vi "FSM Localization.vi"(0 "Signals":T2, 2 "Pressure Controls":T5, 4 "Dialog Indicator":refnum<vi>, 5 "error in (no error)":errorcluster, 6 "Manipulator Dynamics":refnum<vi>, 7 "Unblockage Parameters":T1, 8 "Pressure Levels [KPa]":refnum<vi>, 9 "Test and Offset Controls":T4, 10 "Test Signal Levels":refnum<vi>, 11 "Manipulator Controllers":T3, 13 "Abort":refnum<vi>) -> (15 "Aborted":bool, 16 "Blocked":bool, 19 "error out":errorcluster)   [LabVIEW 2012, in "Autopatcher Daemon.lvlib"]
uses:
  Autopatcher Daemon.lvlib
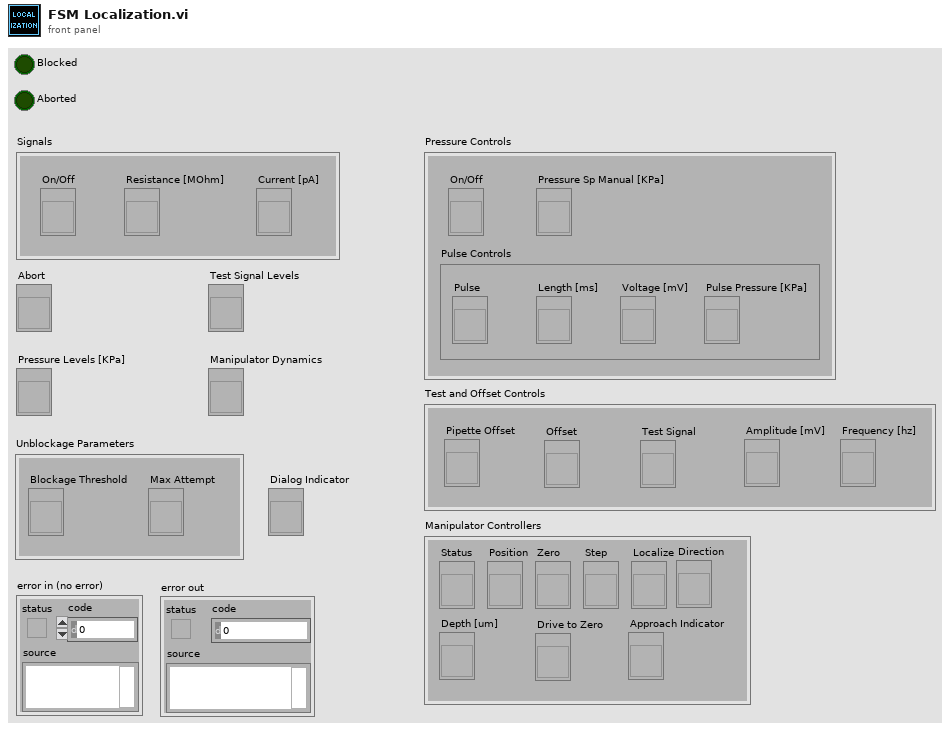
[diagram p1: front panel]
types:
  T1 = cluster{"Blockage Threshold":refnum<vi>, "Max Attempt":refnum<vi>}
  T2 = cluster{"On/Off":refnum<vi>, "Resistance [MOhm]":refnum<vi>, "Current [pA]":refnum<vi>}
  T3 = cluster{"Status":refnum<vi>, "Position":refnum<vi>, "Zero":refnum<vi>, "Step":refnum<vi>, "Localize":refnum<vi>, "Approach Indicator":refnum<vi>, "Depth [um]":refnum<vi>, "Drive to Zero":refnum<vi>, "Direction":refnum<vi>}
  T4 = cluster{"Pipette Offset":refnum<vi>, "Offset":refnum<vi>, "Test Signal":refnum<vi>, "Amplitude [mV]":refnum<vi>, "Frequency [hz]":refnum<vi>}
  T5 = cluster{"On/Off":refnum<vi>, "Pulse Controls":cluster{"Pulse":refnum<vi>, "Length [ms]":refnum<vi>, "Voltage [mV]":refnum<vi>, "Pulse Pressure [KPa]":refnum<vi>}, "Pressure Sp Manual [KPa]":refnum<vi>}
  T6 = cluster{"Seal":cluster{"Amplitude [mV]":i32, "Frequency [hz]":u16}, "Extracellular":cluster{"Amplitude [mV]":i32, "Frequency [hz]":u16}}
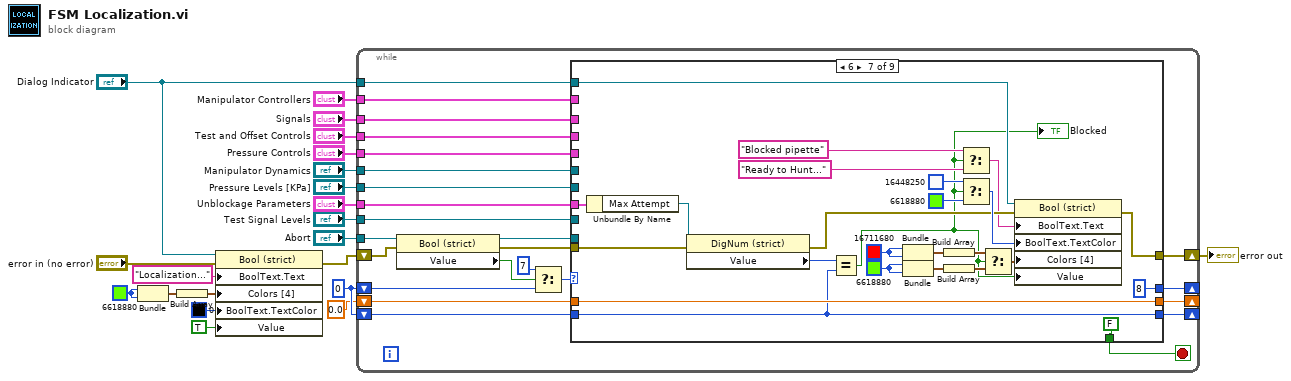
[diagram p0: block diagram]
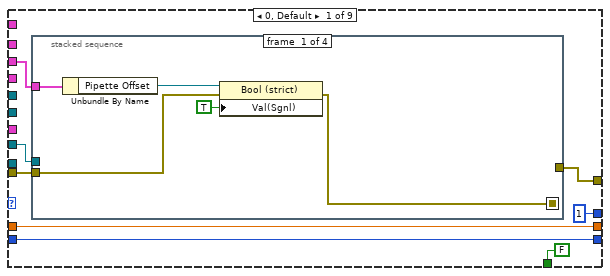
[diagram p2: hidden frame]
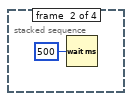
[diagram p3: hidden frame]
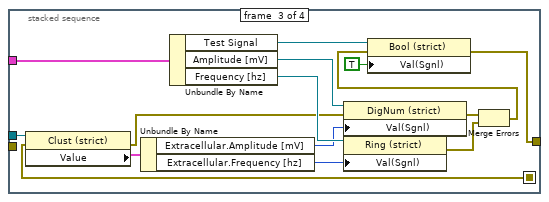
[diagram p4: hidden frame]
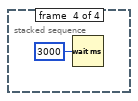
[diagram p5: hidden frame]
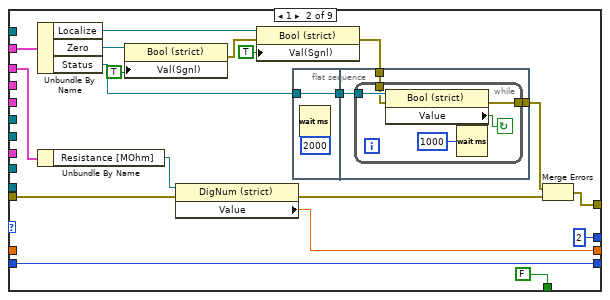
[diagram p6: hidden frame]
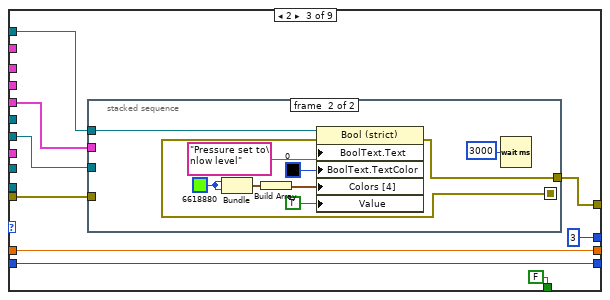
[diagram p7: hidden frame]
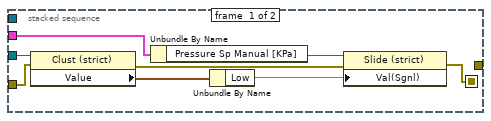
[diagram p8: hidden frame]
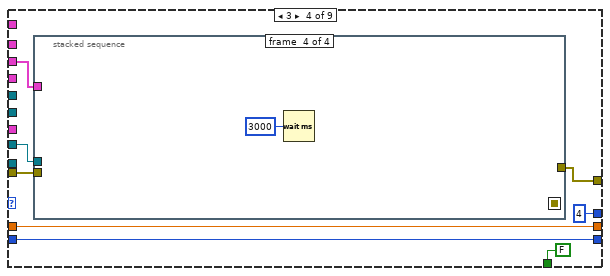
[diagram p9: hidden frame]
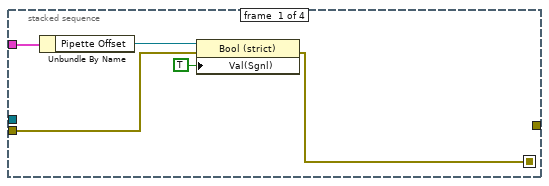
[diagram p10: hidden frame]
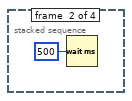
[diagram p11: hidden frame]
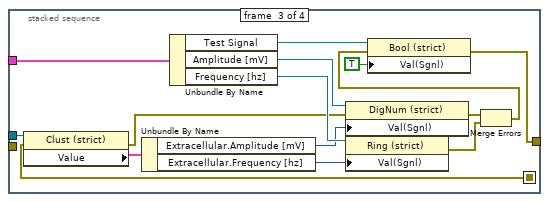
[diagram p12: hidden frame]
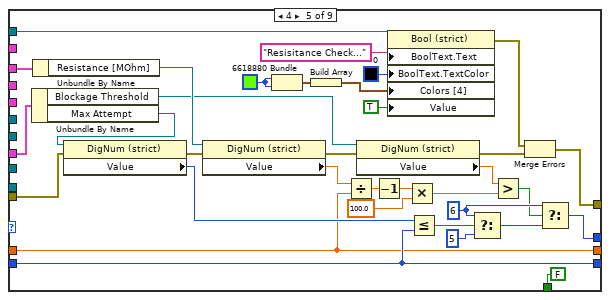
[diagram p13: hidden frame]
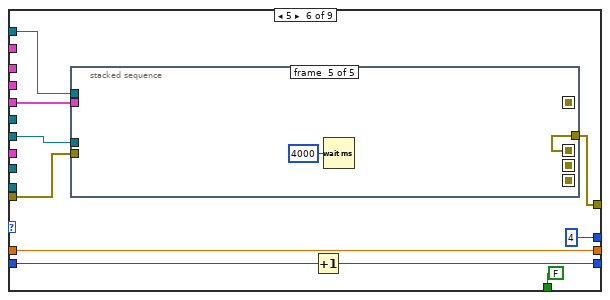
[diagram p14: hidden frame]
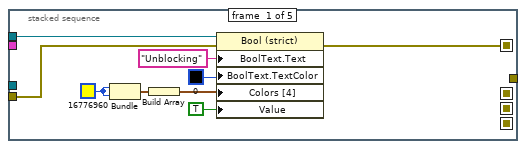
[diagram p15: hidden frame]
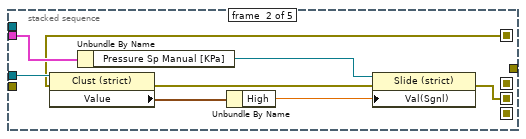
[diagram p16: hidden frame]
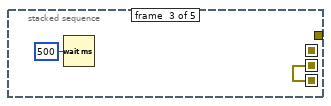
[diagram p17: hidden frame]
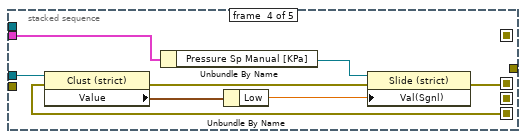
[diagram p18: hidden frame]
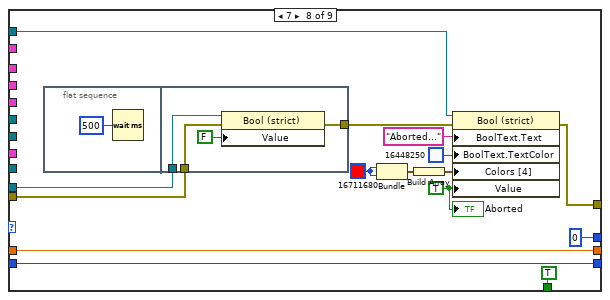
[diagram p19: hidden frame]
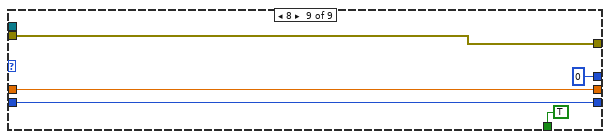
[diagram p20: hidden frame]
diagram:
  w2 = u32 6618880
  w18 = 0
  n1 = Bundle(w2, w2) -> (w6:cluster{u32, u32})  [unwired: 1 in]
  n2 = Build Array(w6) -> (w9:cluster{u32, u32}[])
  n3 = property class="Bool (strict)"(reference="Dialog Indicator", error in="error in (no error)", "BoolText.Text"="Localization..." ("Boolean Text.Text"), "Colors [4]"=w9, "BoolText.TextColor"=u32 0, "Value"=TRUE) -> (error out=w5:errorcluster)  [unwired: 1 out]
  n4 = while {
    shift-right: [w41] -> _
    shift-left: w18 -> [w31]
    shift-right: [w45] -> _
    shift-left: 0.0 ("Value") -> [w44]
    shift-right: [w40] -> _
    shift-left: w18 -> [w39]
    tunnel: "Abort" -> [w33]
    tunnel: "Test Signal Levels" -> [w34]
    tunnel: "Signals" -> [w32]
    tunnel: "Pressure Controls" -> [w37]
    tunnel: "Pressure Levels [KPa]" -> [w36]
    tunnel: "Manipulator Dynamics" -> [w35]
    shift-right: [w42] -> w19
    shift-left: w5 -> [w30]
    tunnel: "Test and Offset Controls" -> [w27]
    tunnel: "Manipulator Controllers" -> [w26]
    tunnel: "Unblockage Parameters" -> [w25]
    tunnel: "Dialog Indicator" -> [w23]
    stop <- w24 stop-if-true
    n5 = property class="Bool (strict)"(reference=w33, error in=w30) -> (reference out=w28:refnum<vi>, error out=w29:errorcluster, "Value"=w22:bool)
    n6 = Select(t=7, s=w22, f=w31) -> (s? t:f=w38:i32)
    n7 = case shown="6" w38 {
      tunnel: [1 2 3 4 w180 4 8 0 0] -> w41
      tunnel: [w52 w84 w112 w138 w177 w204 w258 w274 w284] -> w45
      tunnel: w44 -> [w52 _ w112 w138 w177 w204 w258 w274 w284]
      tunnel: w29 -> [w49 w78 w110 w135 w188 w202 w255 w271 w280]
      tunnel: [w48 w77 w109 w134 w169 w198 w247 w265 w280] -> w42
      tunnel: [w51 w93 w107 w137 w191 w200 w257 w273 w283] -> w40
      tunnel: w39 -> [w51 w93 w107 w137 w191 w199 w257 w273 w283]
      tunnel: w28 -> [_ _ _ _ _ _ _ w270 _]
      tunnel: w34 -> [w46 _ _ w133 _ _ _ _ _]
      tunnel: w32 -> [_ w91 _ _ w194 _ _ _ _]
      tunnel: w37 -> [_ _ w111 _ _ w201 _ _ _]
      tunnel: w36 -> [_ _ w108 _ _ w203 _ _ _]
      tunnel: w35 -> [_ _ _ _ _ _ _ _ _]
      tunnel: w27 -> [w47 _ _ w132 _ _ _ _ _]
      tunnel: w26 -> [_ w85 _ _ _ _ _ _ _]
      tunnel: [FALSE ("x") FALSE ("x") FALSE ("x") FALSE ("x") FALSE ("x") FALSE ("x") FALSE ("x") TRUE ("x") TRUE ("x")] -> w24
      tunnel: w25 -> [_ _ _ _ w186 _ w253 _ _]
      tunnel: w23 -> [_ _ w105 _ w171 w196 w246 w264 _]
      frame 0, Default {
        n8 = stacked-sequence {
          seq-local: [w54 _ _ _] -> [_ _ w62 _]
          tunnel: w46 -> [_ _ w73 _]
          tunnel: w47 -> [w58 _ w65 _]
          tunnel: w49 -> [w55 _ _ _]
          tunnel: [_ _ w61 _] -> w48
          frame #0 {
            n9 = Unbundle By Name(w58) -> ("Pipette Offset"=w56:refnum<vi>)
            n10 = property class="Bool (strict)"(reference=w56, error in=w55, "Val(Sgnl)"=TRUE ("Value (Signaling)")) -> (error out=w54:errorcluster)  [unwired: 1 out]
          }
          frame #1 {
            n11 = Wait (ms)(milliseconds to wait=u32 500) -> ()  [unwired: 1 out]
          }
          frame #2 {
            n12 = property class="Clust (strict)"(reference=w73, error in=w62) -> (error out=w66:errorcluster, "Value"=w74:T6)  [unwired: 1 out]
            n13 = Unbundle By Name(w74) -> ("Extracellular.Amplitude [mV]"=w69:i32, "Extracellular.Frequency [hz]"=w68:u16)
            n14 = Unbundle By Name(w65) -> ("Test Signal"=w67:refnum<vi>, "Amplitude [mV]"=w70:refnum<vi>, "Frequency [hz]"=w71:refnum<vi>)
            n15 = property class="DigNum (strict)"(reference=w70, error in=w66, "Val(Sgnl)"=w69) -> (error out=w63:errorcluster)  [unwired: 1 out]
            n16 = property class="Ring (strict)"(reference=w71, "Val(Sgnl)"=w68) -> (error out=w64:errorcluster)  [unwired: 1 in, 1 out]
            n17 = Merge Errors(w63, w64) -> (w60:errorcluster)
            n18 = property class="Bool (strict)"(reference=w67, error in=w60, "Val(Sgnl)"=TRUE ("Value (Signaling)")) -> (error out=w61:errorcluster)  [unwired: 1 out]
          }
          frame #3 {
            n19 = Wait (ms)(milliseconds to wait=u32 3000) -> ()  [unwired: 1 out]
          }
        }
      }
      frame 1 {
        n20 = Unbundle By Name(w85) -> ("Localize"=w88:refnum<vi>, "Zero"=w86:refnum<vi>, "Status"=w83:refnum<vi>)
        n21 = Unbundle By Name(w91) -> ("Resistance [MOhm]"=w92:refnum<vi>)
        n22 = property class="Bool (strict)"(reference=w86, "Val(Sgnl)"=TRUE ("Value (Signaling)")) -> (error out=w90:errorcluster)  [unwired: 1 in, 1 out]
        n23 = property class="DigNum (strict)"(reference=w92, error in=w78) -> (error out=w80:errorcluster, "Value"=w84:dbl)  [unwired: 1 out]
        n24 = property class="Bool (strict)"(reference=w88, error in=w90, "Val(Sgnl)"=TRUE ("Value (Signaling)")) -> (error out=w82:errorcluster)  [unwired: 1 out]
        n25 = flat-sequence {
          tunnel: w83 -> [w96]
          tunnel: [w96] -> w79
          tunnel: w82 -> [w98]
          tunnel: [w97] -> w81
          tunnel: w79 -> [w99]
          frame #0 {
            n26 = Wait (ms)(milliseconds to wait=u32 2000) -> ()  [unwired: 1 out]
          }
          frame #1 {
            n27 = while {
              tunnel: w99 -> [w103]
              tunnel: [w102] -> w97
              tunnel: w98 -> [w101]
              stop <- w104 continue-if-true
              n28 = property class="Bool (strict)"(reference=w103, error in=w101) -> (error out=w102:errorcluster, "Value"=w104:bool)  [unwired: 1 out]
              n29 = Wait (ms)(milliseconds to wait=u32 1000) -> ()  [unwired: 1 out]
            }
          }
        }
        n30 = Merge Errors(w81, w80) -> (w77:errorcluster)
      }
      frame 2 {
        n31 = stacked-sequence {
          seq-local: [w116 _] -> [_ w125]
          tunnel: w111 -> [w115 _]
          tunnel: w108 -> [w118 _]
          tunnel: w110 -> [w117 _]
          tunnel: [_ w126] -> w109
          tunnel: w105 -> [_ w127]
          frame #0 {
            n32 = property class="Clust (strict)"(reference=w118, error in=w117) -> (error out=w114:errorcluster, "Value"=w119:cluster{"High":dbl, "Low":dbl})  [unwired: 1 out]
            n33 = Unbundle By Name(w115) -> ("Pressure Sp Manual [KPa]"=w120:refnum<vi>)
            n34 = Unbundle By Name(w119) -> ("Low"=w121:dbl)
            n35 = property class="Slide (strict)"(reference=w120, error in=w114, "Val(Sgnl)"=w121) -> (error out=w116:errorcluster)  [unwired: 1 out]
          }
          frame #1 {
            w124 = u32 6618880
            n36 = Bundle(w124, w124) -> (w123:cluster{u32, u32})  [unwired: 1 in]
            n37 = Build Array(w123) -> (w122:cluster{u32, u32}[])
            n38 = property class="Bool (strict)"(reference=w127, error in=w125, "BoolText.Text"="Pressure set to\nlow level" ("Boolean Text.Text"), "BoolText.TextColor"=u32 0, "Colors [4]"=w122, "Value"=TRUE) -> (error out=w126:errorcluster)  [unwired: 1 out]
            n39 = Wait (ms)(milliseconds to wait=u32 3000) -> ()  [unwired: 1 out]
          }
        }
      }
      frame 3 {
        n40 = stacked-sequence {
          seq-local: [w140 _ _ _] -> [_ _ w148 _]
          tunnel: w133 -> [_ _ w159 _]
          tunnel: w132 -> [w144 _ w151 _]
          tunnel: w135 -> [w141 _ _ _]
          tunnel: [_ _ w147 _] -> w134
          frame #0 {
            n41 = Unbundle By Name(w144) -> ("Pipette Offset"=w142:refnum<vi>)
            n42 = property class="Bool (strict)"(reference=w142, error in=w141, "Val(Sgnl)"=TRUE ("Value (Signaling)")) -> (error out=w140:errorcluster)  [unwired: 1 out]
          }
          frame #1 {
            n43 = Wait (ms)(milliseconds to wait=u32 500) -> ()  [unwired: 1 out]
          }
          frame #2 {
            n44 = property class="Clust (strict)"(reference=w159, error in=w148) -> (error out=w152:errorcluster, "Value"=w160:T6)  [unwired: 1 out]
            n45 = Unbundle By Name(w160) -> ("Extracellular.Amplitude [mV]"=w155:i32, "Extracellular.Frequency [hz]"=w154:u16)
            n46 = Unbundle By Name(w151) -> ("Test Signal"=w153:refnum<vi>, "Amplitude [mV]"=w156:refnum<vi>, "Frequency [hz]"=w157:refnum<vi>)
            n47 = property class="DigNum (strict)"(reference=w156, error in=w152, "Val(Sgnl)"=w155) -> (error out=w149:errorcluster)  [unwired: 1 out]
            n48 = property class="Ring (strict)"(reference=w157, "Val(Sgnl)"=w154) -> (error out=w150:errorcluster)  [unwired: 1 in, 1 out]
            n49 = Merge Errors(w149, w150) -> (w146:errorcluster)
            n50 = property class="Bool (strict)"(reference=w153, error in=w146, "Val(Sgnl)"=TRUE ("Value (Signaling)")) -> (error out=w147:errorcluster)  [unwired: 1 out]
          }
          frame #3 {
            n51 = Wait (ms)(milliseconds to wait=u32 3000) -> ()  [unwired: 1 out]
          }
        }
      }
      frame 4 {
        w164 = u32 6618880
        w181 = 6
        n52 = Unbundle By Name(w186) -> ("Blockage Threshold"=w165:refnum<vi>, "Max Attempt"=w185:refnum<vi>)
        n53 = Unbundle By Name(w194) -> ("Resistance [MOhm]"=w195:refnum<vi>)
        n54 = property class="DigNum (strict)"(reference=w185, error in=w188) -> (error out=w189:errorcluster, "Value"=w190:i32)  [unwired: 1 out]
        n55 = property class="DigNum (strict)"(reference=w195, error in=w189) -> (error out=w193:errorcluster, "Value"=w178:dbl)  [unwired: 1 out]
        n56 = Bundle(w164, w164) -> (w163:cluster{u32, u32})  [unwired: 1 in]
        n57 = Build Array(w163) -> (w162:cluster{u32, u32}[])
        n58 = Divide(x=w178, y=w177) -> (x/y=w167:dbl)
        n59 = property class="DigNum (strict)"(reference=w165, error in=w193) -> (error out=w170:errorcluster, "Value"=w192:dbl)  [unwired: 1 out]
        n60 = Decrement(x=w167) -> (x-1=w166:dbl)
        n61 = property class="Bool (strict)"(reference=w171, "BoolText.Text"="Resisitance Check..." ("Boolean Text.Text"), "BoolText.TextColor"=u32 0, "Colors [4]"=w162, "Value"=TRUE) -> (error out=w168:errorcluster)  [unwired: 1 in, 1 out]
        n62 = Multiply(x=w166, y=100.0) -> (x*y=w175:dbl)
        n63 = Less Or Equal?(x=w190, y=w191) -> (x <= y?=w184:bool)
        n64 = Select(t=w181, s=w184, f=5) -> (s? t:f=w183:i32)
        n65 = Greater?(x=w192, y=w175) -> (0:w179:bool)
        n66 = Merge Errors(w168, w170) -> (w169:errorcluster)
        n67 = Select(t=w181, s=w179, f=w183) -> (s? t:f=w180:i32)
      }
      frame 5 {
        n68 = stacked-sequence {
          seq-local: [_ _ w223 _ _] -> [_ _ _ w226 _]
          seq-local: [_ w216 _ _ _] -> [_ _ w223 _ _]
          seq-local: [_ _ _ w225 _] -> [_ _ _ _ w233]
          seq-local: [w209 _ _ _ _] -> [_ w215 _ _ _]
          tunnel: w201 -> [_ w220 _ w227 _]
          tunnel: w203 -> [_ w219 _ w228 _]
          tunnel: w202 -> [w210 _ _ _ _]
          tunnel: [_ _ _ _ w233] -> w198
          tunnel: w196 -> [w212 _ _ _ _]
          frame #0 {
            w208 = u32 16776960
            n69 = Bundle(w208, w208) -> (w207:cluster{u32, u32})  [unwired: 1 in]
            n70 = Build Array(w207) -> (w206:cluster{u32, u32}[])
            n71 = property class="Bool (strict)"(reference=w212, error in=w210, "BoolText.Text"="Unblocking" ("Boolean Text.Text"), "BoolText.TextColor"=u32 0, "Colors [4]"=w206, "Value"=TRUE) -> (error out=w209:errorcluster)  [unwired: 1 out]
          }
          frame #1 {
            n72 = property class="Clust (strict)"(reference=w219, error in=w215) -> (error out=w217:errorcluster, "Value"=w221:cluster{"High":dbl, "Low":dbl})  [unwired: 1 out]
            n73 = Unbundle By Name(w220) -> ("Pressure Sp Manual [KPa]"=w218:refnum<vi>)
            n74 = Unbundle By Name(w221) -> ("High"=w222:dbl)
            n75 = property class="Slide (strict)"(reference=w218, error in=w217, "Val(Sgnl)"=w222) -> (error out=w216:errorcluster)  [unwired: 1 out]
          }
          frame #2 {
            n76 = Wait (ms)(milliseconds to wait=u32 500) -> ()  [unwired: 1 out]
          }
          frame #3 {
            n77 = property class="Clust (strict)"(reference=w228, error in=w226) -> (error out=w229:errorcluster, "Value"=w231:cluster{"High":dbl, "Low":dbl})  [unwired: 1 out]
            n78 = Unbundle By Name(w227) -> ("Pressure Sp Manual [KPa]"=w230:refnum<vi>)
            n79 = Unbundle By Name(w231) -> ("Low"=w232:dbl)
            n80 = property class="Slide (strict)"(reference=w230, error in=w229, "Val(Sgnl)"=w232) -> (error out=w225:errorcluster)  [unwired: 1 out]
          }
          frame #4 {
            n81 = Wait (ms)(milliseconds to wait=u32 4000) -> ()  [unwired: 1 out]
          }
        }
        n82 = Increment(x=w199) -> (x+1=w200:i32)
      }
      frame 6 {
        w239 = u32 6618880
        w242 = u32 16711680
        n83 = Unbundle By Name(w253) -> ("Max Attempt"=w252:refnum<vi>)
        n84 = property class="DigNum (strict)"(reference=w252, error in=w255) -> (error out=w248:errorcluster, "Value"=w256:i32)  [unwired: 1 out]
        n85 = Equal?(x=w256, y=w257) -> (x = y?=w235:bool)
        "Blocked" <- w235
        n86 = Bundle(w242, w242) -> (w241:cluster{u32, u32})  [unwired: 1 in]
        n87 = Bundle(w239, w239) -> (w238:cluster{u32, u32})  [unwired: 1 in]
        n88 = Build Array(w241) -> (w240:cluster{u32, u32}[])
        n89 = Build Array(w238) -> (w237:cluster{u32, u32}[])
        n90 = Select(t="Blocked pipette" ("Boolean Text.Text"), s=w235, f="Ready to Hunt..." ("Boolean Text.Text")) -> (s? t:f=w245:string)
        n91 = Select(t=u32 16448250, s=w235, f=u32 6618880) -> (s? t:f=w249:u32)
        n92 = Select(t=w240, s=w235, f=w237) -> (s? t:f=w236:cluster{u32, u32}[])
        n93 = property class="Bool (strict)"(reference=w246, error in=w248, "BoolText.Text"=w245, "BoolText.TextColor"=w249, "Colors [4]"=w236, "Value"=w235) -> (error out=w247:errorcluster)  [unwired: 1 out]
      }
      frame 7 {
        w263 = u32 16711680
        w260 = TRUE ("Value")
        n94 = flat-sequence {
          tunnel: [w278] -> w266
          tunnel: w271 -> [w277]
          tunnel: w270 -> [w276]
          frame #0 {
            n95 = Wait (ms)(milliseconds to wait=u32 500) -> ()  [unwired: 1 out]
          }
          frame #1 {
            n96 = property class="Bool (strict)"(reference=w276, error in=w277, "Value"=FALSE) -> (error out=w278:errorcluster)  [unwired: 1 out]
          }
        }
        n97 = Bundle(w263, w263) -> (w262:cluster{u32, u32})  [unwired: 1 in]
        n98 = Build Array(w262) -> (w261:cluster{u32, u32}[])
        n99 = property class="Bool (strict)"(reference=w264, error in=w266, "BoolText.Text"="Aborted..." ("Boolean Text.Text"), "BoolText.TextColor"=u32 16448250, "Colors [4]"=w261, "Value"=w260) -> (error out=w265:errorcluster)  [unwired: 1 out]
        "Aborted" <- w260
      }
      frame 8 {
      }
    }
  }
  "error out" <- w19
